vi "Write a.vi"(9 "a":dbl, 11 "Dual in":refnum<class "Dual.lvclass">) -> (3 "Dual out":refnum<class "Dual.lvclass">)   [LabVIEW 2020, in "Automatic Differentiation.lvlib" / "Dual.lvclass"]
uses:
  Dual.lvclass
  Dual.lvclass/Dual.ctl
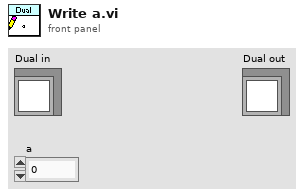
[diagram p1: front panel]
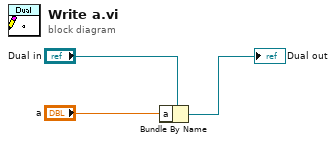
[diagram p0: block diagram]
diagram:
  n1 = Bundle By Name(cluster="Dual in", "a"="a") -> (→"Dual out":refnum<class "Dual.lvclass">)
